vi "Lista.vi"(3 "error in (no error)":errorcluster) -> (0 "error out":errorcluster, 1 "Password":string, 2 "Login":string)   [LabVIEW 2014]
panel:
  out "String 2":string
  in  "String":string="Por favor introduzca su contraseña"
  in  "OK Button 12":bool
  in  "OK Button 11":bool
  out "Numeric":i32
  out "Array 2":u8[](array[numeric]) format="%x"
  out "D4":string
  out "D3":string
  out "D2":string
  out "D1":string
  in  "OK Button 10":bool
  in  "OK Button 9":bool
  in  "OK Button 8":bool
  in  "OK Button 7":bool
  in  "OK Button 6":bool
  in  "OK Button 5":bool
  in  "OK Button 4":bool
  in  "OK Button 3":bool
  in  "OK Button 2":bool
  in  "OK Button":bool
  out "element":i32
  out "size(s)":i32
  in  "Listbox":i32[](listbox)
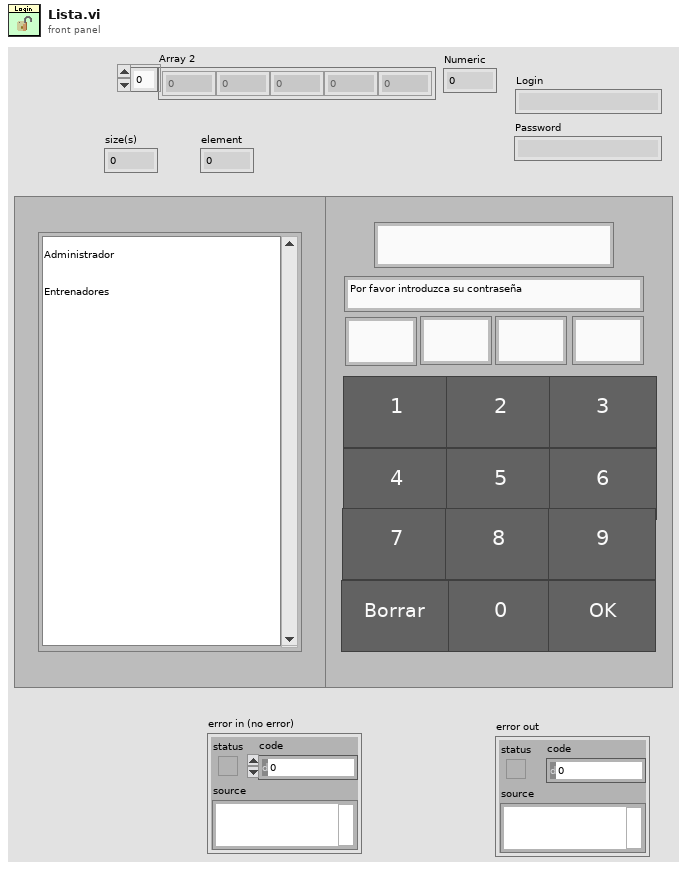
[diagram p1: front panel]
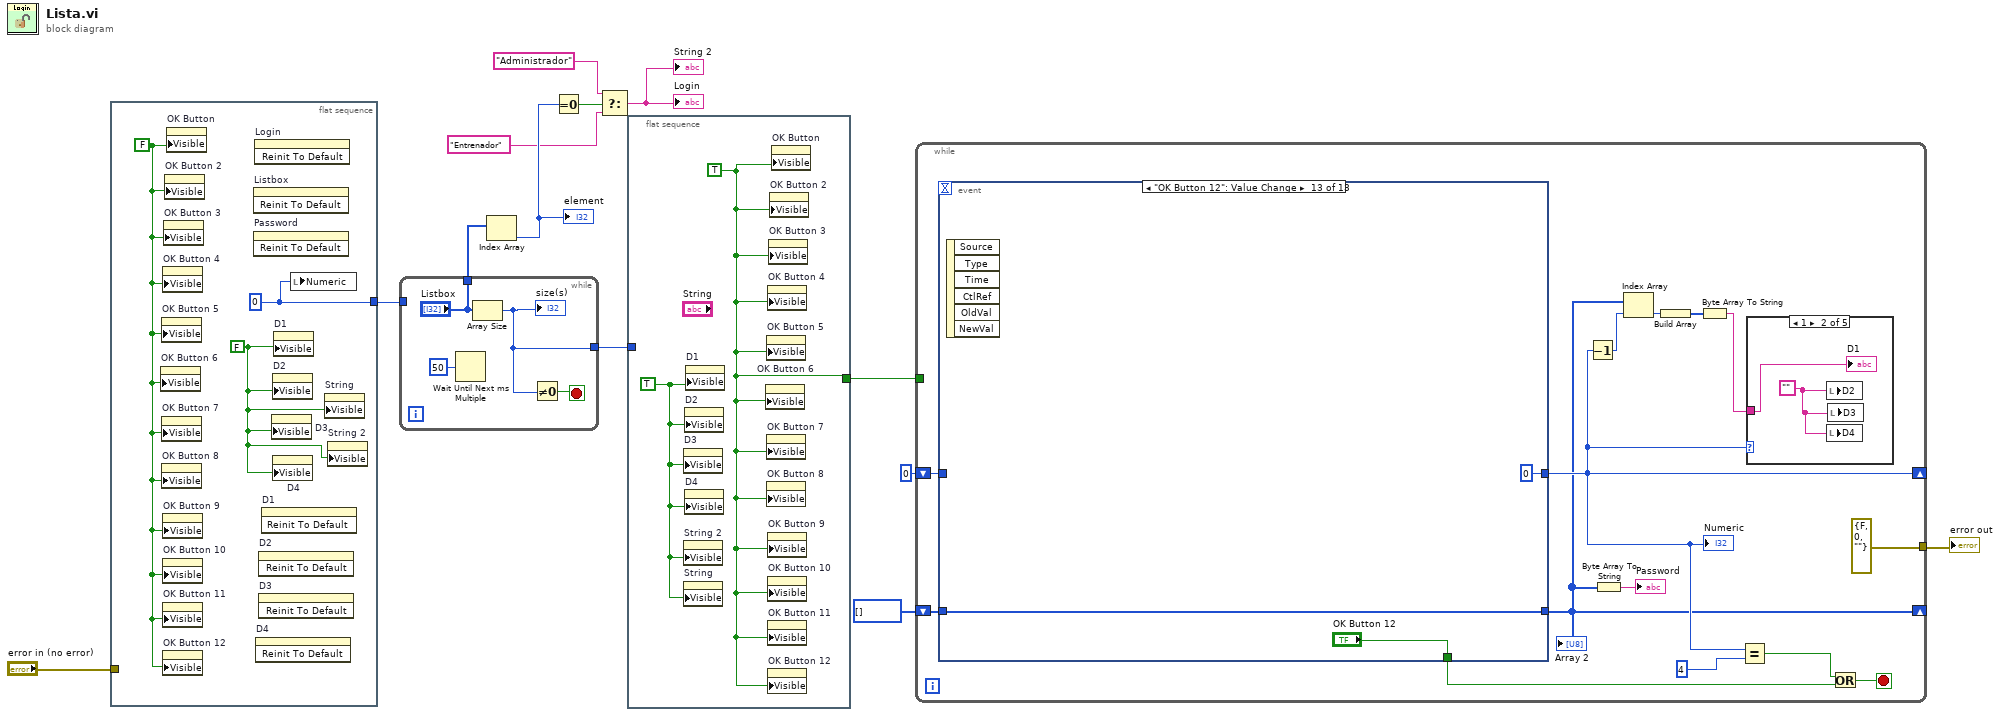
[diagram p0: block diagram]
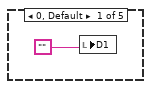
[diagram p2: hidden frame]
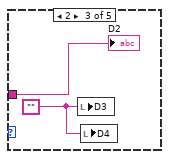
[diagram p3: hidden frame]
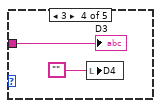
[diagram p4: hidden frame]
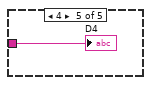
[diagram p5: hidden frame]
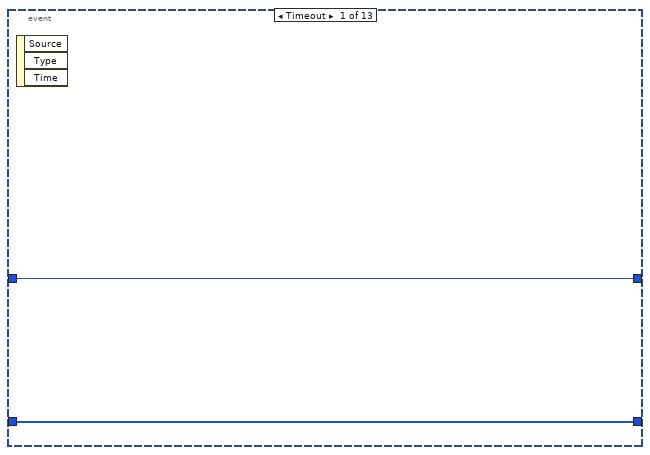
[diagram p6: hidden frame]
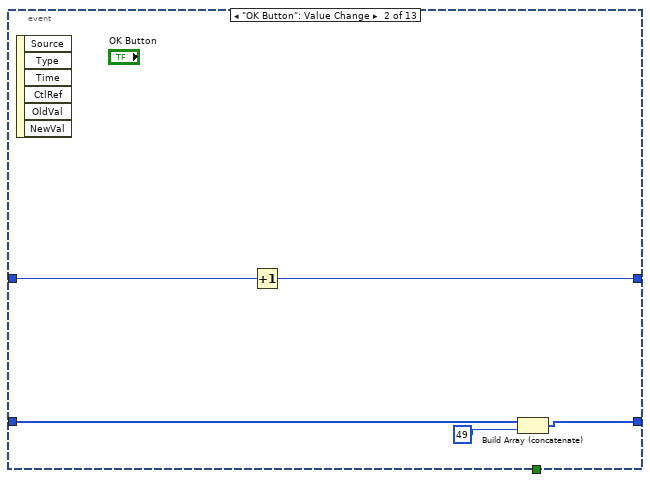
[diagram p7: hidden frame]
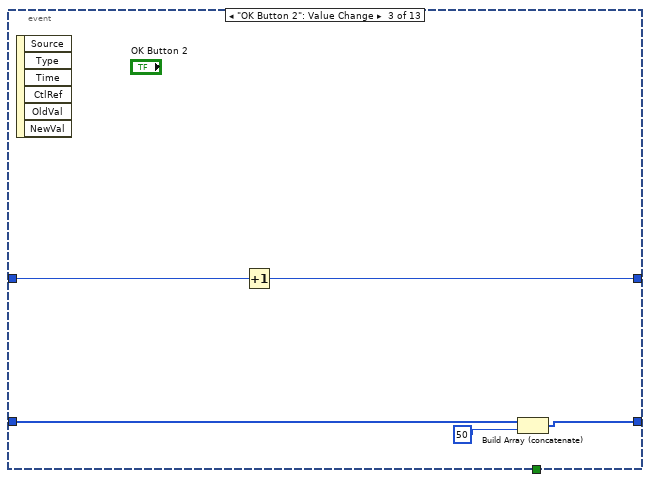
[diagram p8: hidden frame]
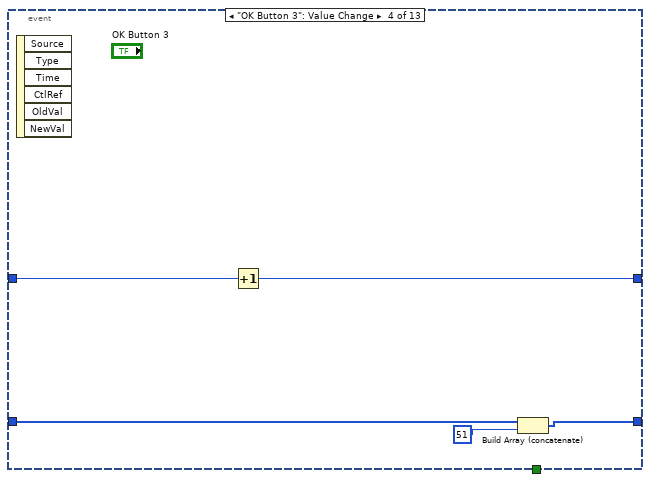
[diagram p9: hidden frame]
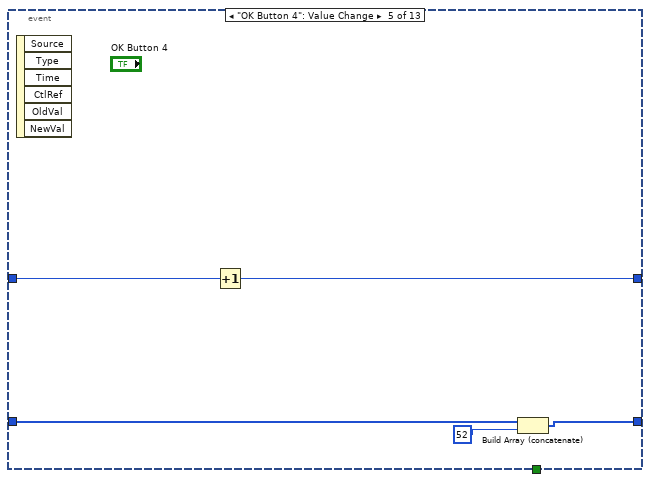
[diagram p10: hidden frame]
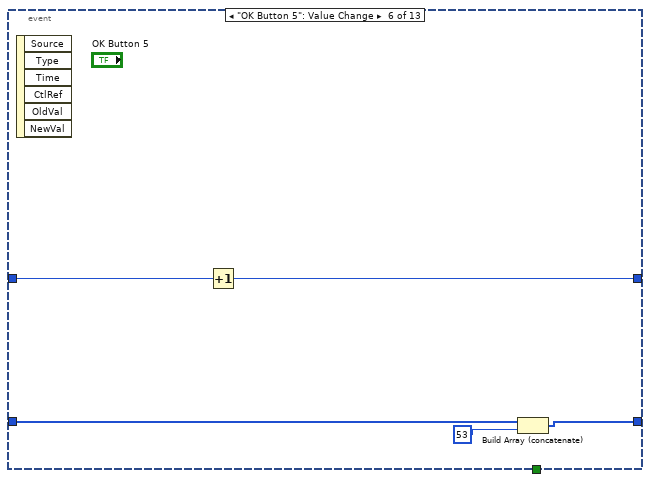
[diagram p11: hidden frame]
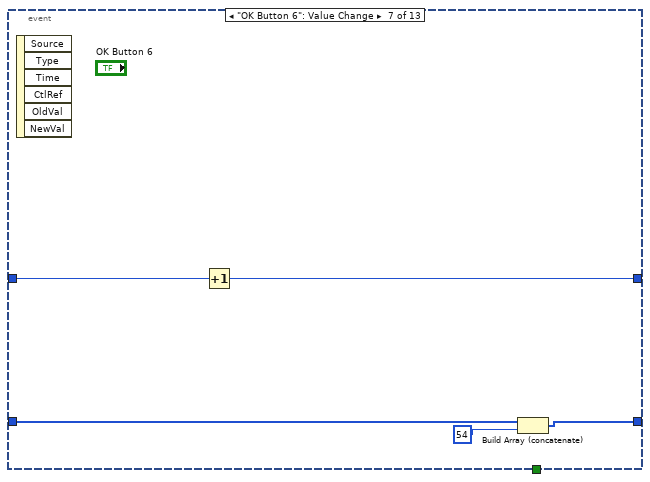
[diagram p12: hidden frame]
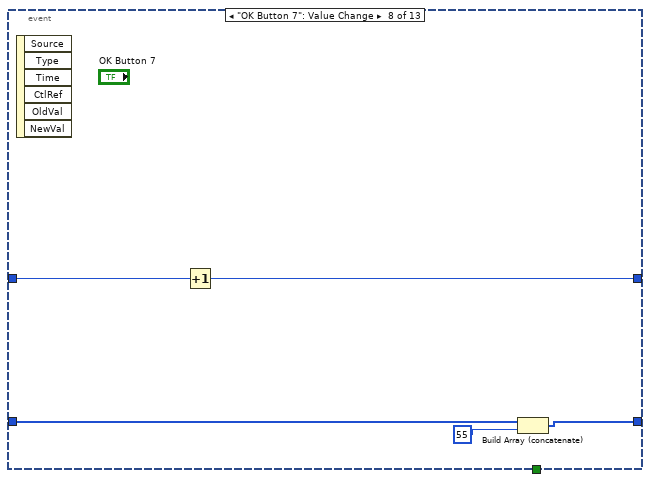
[diagram p13: hidden frame]
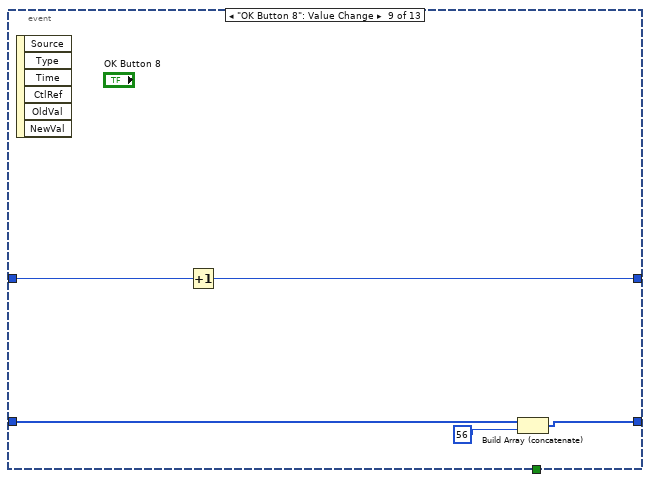
[diagram p14: hidden frame]
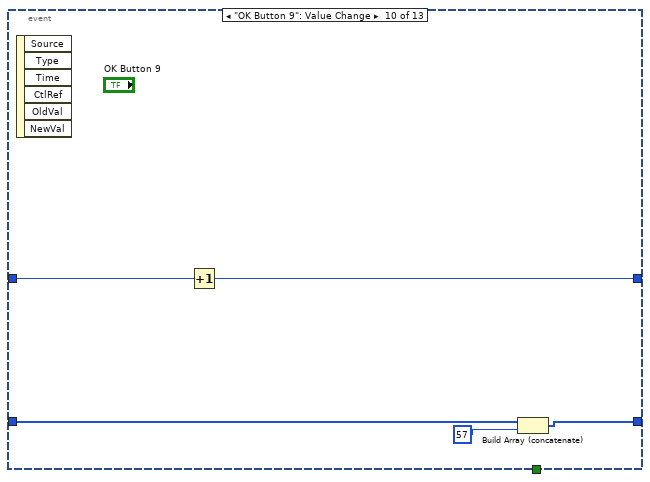
[diagram p15: hidden frame]
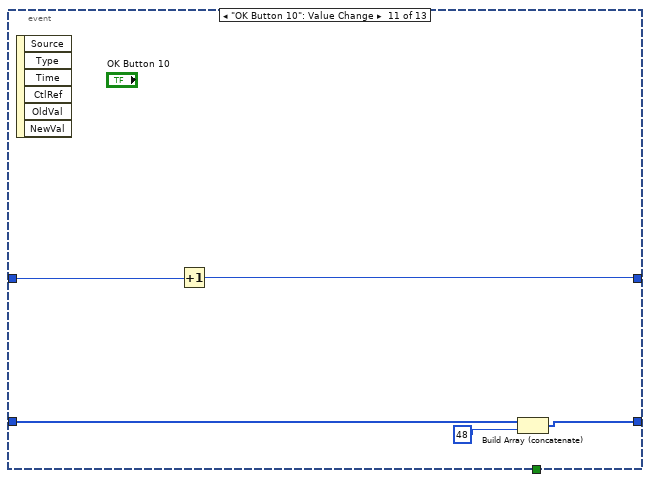
[diagram p16: hidden frame]
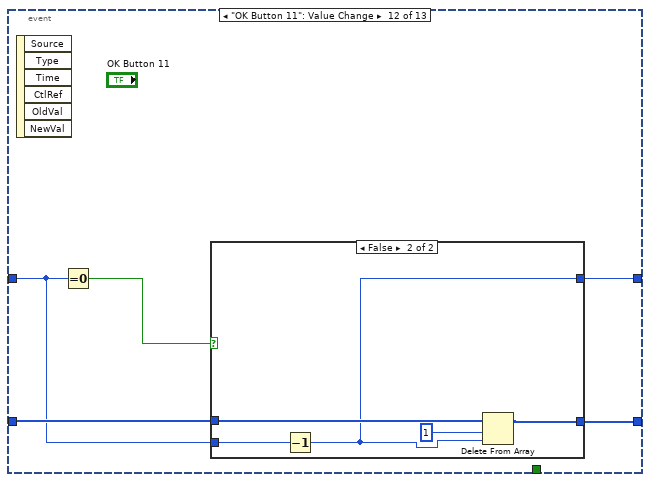
[diagram p17: hidden frame]
diagram:
  n1 = flat-sequence {
    tunnel: [w15] -> w6
    tunnel: "error in (no error)" -> [_]
    frame #0 {
      w14 = FALSE
      w16 = FALSE
      w15 = 0 ("Numeric")
      n2 = property on="OK Button 6" class="Bool"("Visible"=w16) -> ()  [unwired: 2 in, 2 out]
      n3 = property on="OK Button 5" class="Bool"("Visible"=w16) -> ()  [unwired: 2 in, 2 out]
      n4 = property on="OK Button 7" class="Bool"("Visible"=w16) -> ()  [unwired: 2 in, 2 out]
      n5 = property on="OK Button 8" class="Bool"("Visible"=w16) -> ()  [unwired: 2 in, 2 out]
      n6 = property on="OK Button 4" class="Bool"("Visible"=w16) -> ()  [unwired: 2 in, 2 out]
      n7 = property on="OK Button 9" class="Bool"("Visible"=w16) -> ()  [unwired: 2 in, 2 out]
      n8 = property on="OK Button 10" class="Bool"("Visible"=w16) -> ()  [unwired: 2 in, 2 out]
      n9 = property on="OK Button 11" class="Bool"("Visible"=w16) -> ()  [unwired: 2 in, 2 out]
      n10 = property on="OK Button 12" class="Bool"("Visible"=w16) -> ()  [unwired: 2 in, 2 out]
      n11 = property on="OK Button 3" class="Bool"("Visible"=w16) -> ()  [unwired: 2 in, 2 out]
      n12 = property on="OK Button 2" class="Bool"("Visible"=w16) -> ()  [unwired: 2 in, 2 out]
      n13 = property on="OK Button" class="Bool"("Visible"=w16) -> ()  [unwired: 2 in, 2 out]
      n14 = invoke on="Listbox" class="LstBox (strict)" method="Reinit To Default"() -> ()  [unwired: 3 in, 3 out]
      n15 = invoke on="Password" class="Str" method="Reinit To Default"() -> ()  [unwired: 3 in, 3 out]
      n16 = invoke on="Login" class="Str" method="Reinit To Default"() -> ()  [unwired: 3 in, 3 out]
      n17 = invoke on="D4" class="Str" method="Reinit To Default"() -> ()  [unwired: 3 in, 3 out]
      n18 = invoke on="D2" class="Str" method="Reinit To Default"() -> ()  [unwired: 3 in, 3 out]
      n19 = invoke on="D3" class="Str" method="Reinit To Default"() -> ()  [unwired: 3 in, 3 out]
      n20 = invoke on="D1" class="Str" method="Reinit To Default"() -> ()  [unwired: 3 in, 3 out]
      n21 = property on="D3" class="Str"("Visible"=w14) -> ()  [unwired: 2 in, 2 out]
      n22 = property on="D2" class="Str"("Visible"=w14) -> ()  [unwired: 2 in, 2 out]
      n23 = property on="D4" class="Str"("Visible"=w14) -> ()  [unwired: 2 in, 2 out]
      n24 = property on="D1" class="Str"("Visible"=w14) -> ()  [unwired: 2 in, 2 out]
      n25 = local write "Numeric"(w15) -> ()
      n26 = property on="String" class="Str"("Visible"=w14) -> ()  [unwired: 2 in, 2 out]
      n27 = property on="String 2" class="Str"("Visible"=w14) -> ()  [unwired: 2 in, 2 out]
    }
  }
  n28 = while {
    tunnel: ["Listbox"] -> w13
    tunnel: w6 -> [_]
    tunnel: [w17] -> w4
    stop <- w19 stop-if-true
    n29 = Wait Until Next ms Multiple(millisecond multiple=u32 50) -> ()  [unwired: 1 out]
    n30 = Array Size(array="Listbox") -> (size(s)=w17:i32)
    "size(s)" <- w17
    n31 = Not Equal To 0?(x=w17) -> (x != 0?=w19:bool)
  }
  n32 = Index Array(array=w13) -> (element=w10:i32)  [unwired: 1 in]
  "element" <- w10
  n33 = Equal To 0?(x=w10) -> (x = 0?=w9:bool)
  n34 = Select(t="Administrador", s=w9, f="Entrenador") -> (s? t:f=→"Login" →"String 2":string)
  n35 = flat-sequence {
    tunnel: [w22] -> w5
    tunnel: w4 -> [_]
    frame #0 {
      w21 = TRUE
      w22 = TRUE
      n36 = property on="D3" class="Str"("Visible"=w21) -> ()  [unwired: 2 in, 2 out]
      n37 = property on="String 2" class="Str"("Visible"=w21) -> ()  [unwired: 2 in, 2 out]
      n38 = property on="String" class="Str"("Visible"=w21) -> ()  [unwired: 2 in, 2 out]
      n39 = property on="D2" class="Str"("Visible"=w21) -> ()  [unwired: 2 in, 2 out]
      n40 = property on="D4" class="Str"("Visible"=w21) -> ()  [unwired: 2 in, 2 out]
      n41 = property on="D1" class="Str"("Visible"=w21) -> ()  [unwired: 2 in, 2 out]
      n42 = property on="OK Button 6" class="Bool"("Visible"=w22) -> ()  [unwired: 2 in, 2 out]
      n43 = property on="OK Button 5" class="Bool"("Visible"=w22) -> ()  [unwired: 2 in, 2 out]
      n44 = property on="OK Button 7" class="Bool"("Visible"=w22) -> ()  [unwired: 2 in, 2 out]
      n45 = property on="OK Button 8" class="Bool"("Visible"=w22) -> ()  [unwired: 2 in, 2 out]
      n46 = property on="OK Button 4" class="Bool"("Visible"=w22) -> ()  [unwired: 2 in, 2 out]
      n47 = property on="OK Button 9" class="Bool"("Visible"=w22) -> ()  [unwired: 2 in, 2 out]
      n48 = property on="OK Button 10" class="Bool"("Visible"=w22) -> ()  [unwired: 2 in, 2 out]
      n49 = property on="OK Button 11" class="Bool"("Visible"=w22) -> ()  [unwired: 2 in, 2 out]
      n50 = property on="OK Button 12" class="Bool"("Visible"=w22) -> ()  [unwired: 2 in, 2 out]
      n51 = property on="OK Button 3" class="Bool"("Visible"=w22) -> ()  [unwired: 2 in, 2 out]
      n52 = property on="OK Button 2" class="Bool"("Visible"=w22) -> ()  [unwired: 2 in, 2 out]
      n53 = property on="OK Button" class="Bool"("Visible"=w22) -> ()  [unwired: 2 in, 2 out]
    }
  }
  n54 = while {
    shift-right: [w24] -> _
    shift-left: u8[] [] -> [w36]
    shift-right: [w26] -> _
    shift-left: 0 -> [w35]
    tunnel: w5 -> [_]
    tunnel: [errorcluster {"status"=FALSE, "code"=0, "source"=""} ("error out")] -> w1
    stop <- w29 stop-if-true
    n55 = event shown="[12] \"OK Button 12\": Value Change" {
      selector: _ -> [_ _ _ _ _ _ _ _ _ _ _ _ _]
      dyn-events: _ -> [_ _ _ _ _ _ _ _ _ _ _ _ _]
      timeout: _ -> [_ _ _ _ _ _ _ _ _ _ _ _ _]
      tunnel: [w46 w51 w56 w61 w66 w71 w76 w81 w86 w91 w96 w101 w111] -> w24
      tunnel: w36 -> [w46 w50 w55 w60 w65 w70 w75 w80 w85 w90 w95 w100 w111]
      tunnel: [_ _ _ _ _ _ _ _ _ _ _ _ "OK Button 12"] -> w28
      tunnel: w35 -> [w45 w48 w53 w57 w63 w67 w73 w78 w83 w88 w93 w99 _]
      tunnel: [w45 w47 w52 w58 w62 w68 w72 w77 w82 w87 w92 w97 0] -> w26
      event Timeout {
        n56 = event-data() -> ()  [unwired: 1 in, 3 out]
      }
      event "OK Button": Value Change {
        n57 = event-data() -> ()  [unwired: 1 in, 6 out]
        n58 = Increment(x=w48) -> (x+1=w47:i32)
        n59 = Build Array (concatenate)(w50, u8 49) -> (w51:u8[])
      }
      event "OK Button 2": Value Change {
        n60 = event-data() -> ()  [unwired: 1 in, 6 out]
        n61 = Increment(x=w53) -> (x+1=w52:i32)
        n62 = Build Array (concatenate)(w55, u8 50) -> (w56:u8[])
      }
      event "OK Button 3": Value Change {
        n63 = event-data() -> ()  [unwired: 1 in, 6 out]
        n64 = Increment(x=w57) -> (x+1=w58:i32)
        n65 = Build Array (concatenate)(w60, u8 51) -> (w61:u8[])
      }
      event "OK Button 4": Value Change {
        n66 = event-data() -> ()  [unwired: 1 in, 6 out]
        n67 = Increment(x=w63) -> (x+1=w62:i32)
        n68 = Build Array (concatenate)(w65, u8 52) -> (w66:u8[])
      }
      event "OK Button 5": Value Change {
        n69 = event-data() -> ()  [unwired: 1 in, 6 out]
        n70 = Increment(x=w67) -> (x+1=w68:i32)
        n71 = Build Array (concatenate)(w70, u8 53) -> (w71:u8[])
      }
      event "OK Button 6": Value Change {
        n72 = event-data() -> ()  [unwired: 1 in, 6 out]
        n73 = Increment(x=w73) -> (x+1=w72:i32)
        n74 = Build Array (concatenate)(w75, u8 54) -> (w76:u8[])
      }
      event "OK Button 7": Value Change {
        n75 = event-data() -> ()  [unwired: 1 in, 6 out]
        n76 = Increment(x=w78) -> (x+1=w77:i32)
        n77 = Build Array (concatenate)(w80, u8 55) -> (w81:u8[])
      }
      event "OK Button 8": Value Change {
        n78 = event-data() -> ()  [unwired: 1 in, 6 out]
        n79 = Increment(x=w83) -> (x+1=w82:i32)
        n80 = Build Array (concatenate)(w85, u8 56) -> (w86:u8[])
      }
      event "OK Button 9": Value Change {
        n81 = event-data() -> ()  [unwired: 1 in, 6 out]
        n82 = Increment(x=w88) -> (x+1=w87:i32)
        n83 = Build Array (concatenate)(w90, u8 57) -> (w91:u8[])
      }
      event "OK Button 10": Value Change {
        n84 = event-data() -> ()  [unwired: 1 in, 6 out]
        n85 = Increment(x=w93) -> (x+1=w92:i32)
        n86 = Build Array (concatenate)(w95, u8 48) -> (w96:u8[])
      }
      event "OK Button 11": Value Change {
        n87 = event-data() -> ()  [unwired: 1 in, 6 out]
        n88 = Equal To 0?(x=w99) -> (x = 0?=w98:bool)
        n89 = case shown="False" w98 {
          tunnel: [w102 w108] -> w101
          tunnel: w100 -> [w102 w107]
          tunnel: w99 -> [w103 w105]
          tunnel: [w103 w104] -> w97
          frame True {
          }
          frame False {
            n90 = Decrement(x=w105) -> (x-1=w104:i32)
            n91 = Delete From Array(array=w107, length=1, index=w104) -> (array with subset deleted=w108:u8[])  [unwired: 1 out]
          }
        }
      }
      event "OK Button 12": Value Change {
        n92 = event-data() -> ()  [unwired: 1 in, 6 out]
      }
    }
    "Array 2" <- w24
    "Numeric" <- w26
    n93 = Decrement(x=w26) -> (x-1=w31:i32)
    n94 = Byte Array To String(unsigned byte array=w24) -> (string=→"Password":string)
    n95 = Index Array(array=w24, index=w31) -> (element=w33:u8)
    n96 = Build Array(w33) -> (w32:u8[])
    n97 = Byte Array To String(unsigned byte array=w32) -> (string=w30:string)
    n98 = Equal?(x=w26, y=4) -> (x = y?=w27:bool)
    n99 = case shown="1" w26 {
      tunnel: w30 -> [_ w39 w41 w43 w44]
      frame 0, Default {
        n100 = local write "D1"("") -> ()
      }
      frame 1 {
        w38 = ""
        n101 = local write "D2"(w38) -> ()
        n102 = local write "D4"(w38) -> ()
        n103 = local write "D3"(w38) -> ()
        "D1" <- w39
      }
      frame 2 {
        w40 = ""
        n104 = local write "D3"(w40) -> ()
        n105 = local write "D4"(w40) -> ()
        "D2" <- w41
      }
      frame 3 {
        n106 = local write "D4"("") -> ()
        "D3" <- w43
      }
      frame 4 {
        "D4" <- w44
      }
    }
    n107 = Or(x=w27, y=w28) -> (x .or. y?=w29:bool)
  }
  "error out" <- w1
